vi "LINC Parse Text Command.vi"(8 "error in (no error)":errorcluster, 9 "string command":string, 10 "target name":string) -> (0 "error out":errorcluster, 1 "member data":string[](array[string]), 2 "member names":string[](array[string]), 3 "packet name":string, 5 "member types":string[](array[string]))   [LabVIEW 2018, in "STEPkgDriver_LINC.lvlib"]
uses:
  STEPkgDriver_LINC.lvlib
  LINC Global Mode.ctl
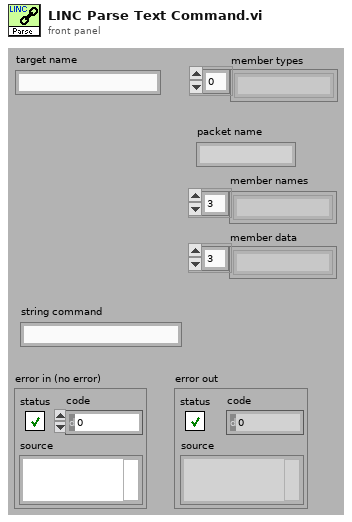
[diagram p1: front panel]
types:
  T1 = typedef "STEPkgDriver_LINC.lvlib/LINC Global Mode.ctl" = enum16{"INIT", "CLEAR", "ADD_PKT_HDR", "ADD_PKT", "GET_PKT_NAMES", "GET_PKT_DESC", "GET_PKT_HDR", "GET_PKT", "SET_PKT", "SET_DATA", "SIM_EN", "SIM_DS"}
  T2 = typedef "STEPkgDriver_LINC.lvlib/LINC Format Prototype.ctl" = cluster{"type":string, "bit offset":i32, "bit size":i32, "format":string, "unit":string, "description":string, "state values":i64[], "states":string[], "max":string, "min":string, "default":string, "array":bool, "bit element size":i32, "poly bound":dbl[], "poly scale":cluster{"coefficients":dbl[]}[], "labview size":i32, "simulate":bool, "ID":bool, "required":bool}
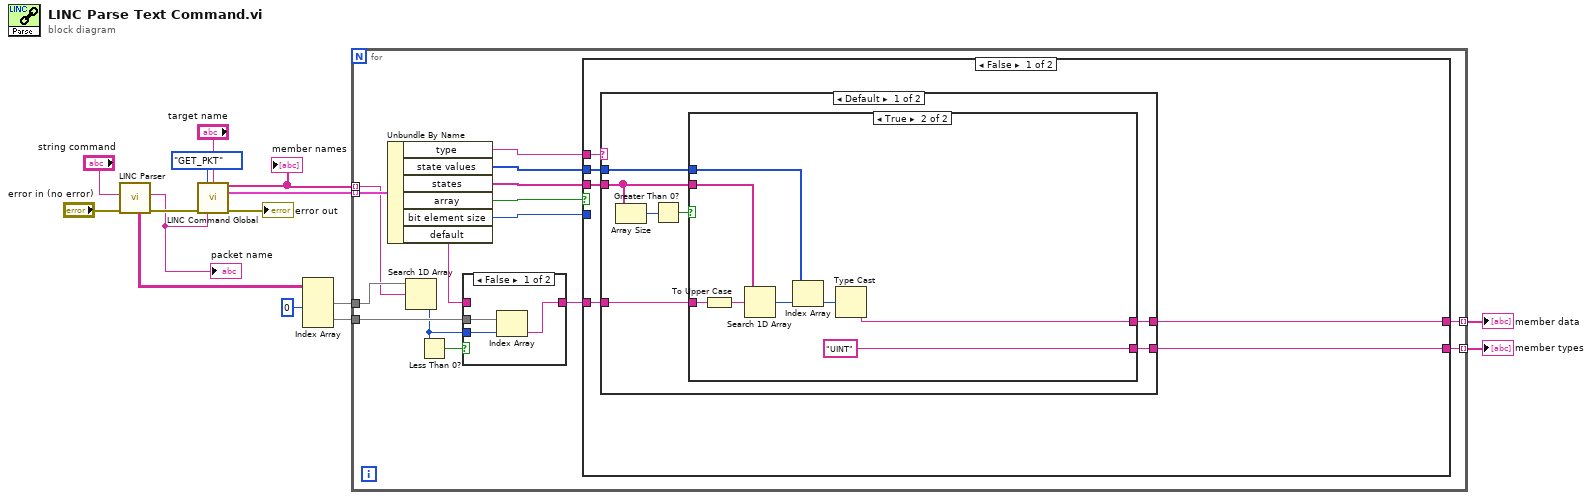
[diagram p0: block diagram]
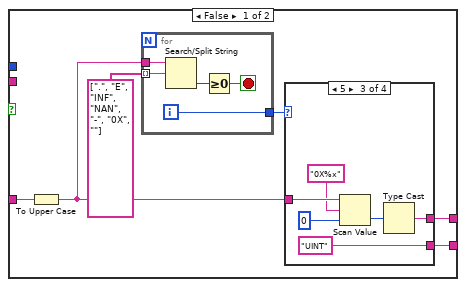
[diagram p3: hidden frame]
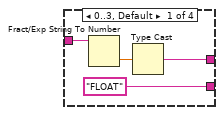
[diagram p4: hidden frame]
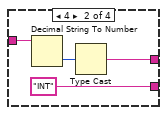
[diagram p5: hidden frame]
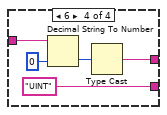
[diagram p6: hidden frame]
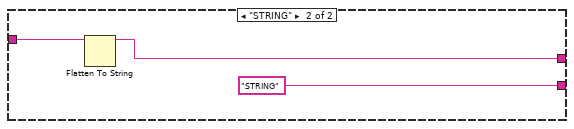
[diagram p7: hidden frame]
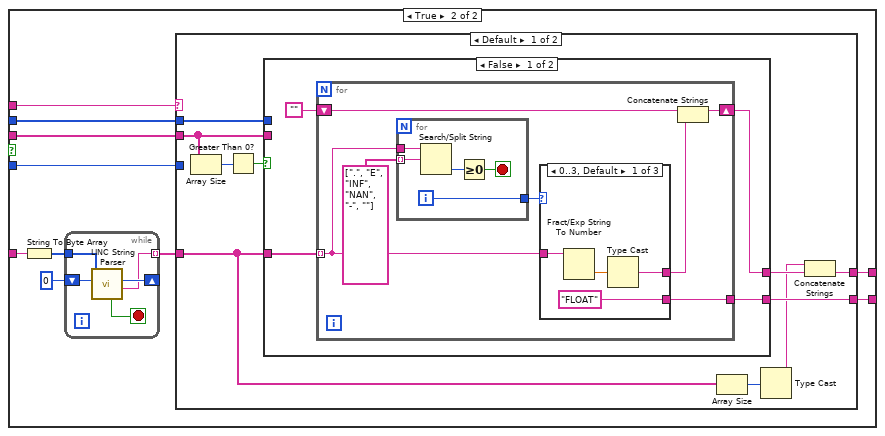
[diagram p8: hidden frame]
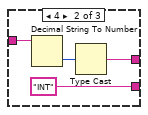
[diagram p9: hidden frame]
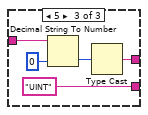
[diagram p10: hidden frame]
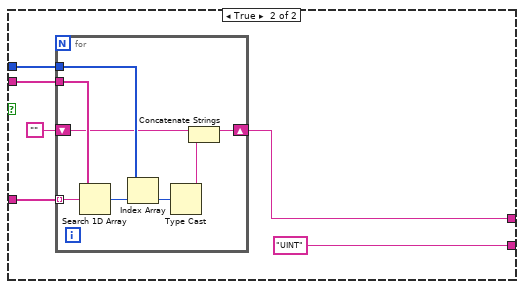
[diagram p11: hidden frame]
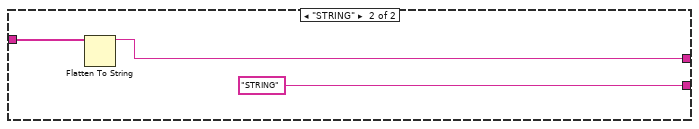
[diagram p12: hidden frame]
diagram:
  n1 = call "LINC Parser.vi"("error in (no error)"="error in (no error)", "command in"="string command") -> ("error out"=w4:errorcluster, "command"=w1:string, "command arguments"=w9:string[][])  [unwired: 7 in]
  "packet name" <- w1
  n2 = call "LINC Command Global.vi"("mode"=LINC_Global_Mode."GET_PKT", "target name"="target name", "error in (no error)"=w4, "packet name"=w1) -> ("values out"=w12:string[], "item formats out"=w11:T2[], "error out"=→"error out":errorcluster)  [unwired: 7 in, 2 out]
  "member names" <- w12
  n3 = Index Array(array=w9, index (col) #1=0 ("index")) -> (element #1=w8:string[], element #2=w7:string[])  [unwired: 3 in]
  n4 = for {
    tunnel: w11 -> [w26] mode=indexing
    tunnel: w12 -> [w24] mode=indexing
    tunnel: w8 -> [w25]
    tunnel: w7 -> [w23]
    tunnel: [w21] -> w6 mode=indexing
    tunnel: [w20] -> w5 mode=indexing
    n5 = Unbundle By Name(w26) -> ("type"=w29:string, "state values"=w28:i64[], "states"=w27:string[], "array"=w30:bool, "bit element size"=w16:i32, "default"=w17:string)
    n6 = Search 1D Array(1D array=w25, element=w24) -> (index of element=w19:i32)  [unwired: 1 in]
    n7 = Less Than 0?(x=w19) -> (x < 0?=w18:bool)
    n8 = case shown="False" w18 {
      tunnel: w23 -> [w33 _]
      tunnel: [w32 w34] -> w22
      tunnel: w19 -> [w31 _]
      tunnel: w17 -> [_ w34]
      frame False {
        n9 = Index Array(array=w33, index=w31) -> (element=w32:string)
      }
      frame True {
      }
    }
    n10 = case shown="False" w30 {
      tunnel: w29 -> [w40 w98]
      tunnel: w22 -> [w39 w93]
      tunnel: w28 -> [w38 w97]
      tunnel: w27 -> [w37 w96]
      tunnel: [w36 w90] -> w20
      tunnel: [w35 w89] -> w21
      tunnel: w16 -> [_ w92]
      frame False {
        n11 = case shown="Default" w40 {
          tunnel: w39 -> [w46 w87]
          tunnel: w38 -> [w43 _]
          tunnel: w37 -> [w44 _]
          tunnel: [w41 w86] -> w36
          tunnel: [w42 "STRING" ("new element/subarray")] -> w35
          frame Default {
            n12 = Array Size(array=w44) -> (size(s)=w47:i32)
            n13 = Greater Than 0?(x=w47) -> (x > 0?=w45:bool)
            n14 = case shown="True" w45 {
              tunnel: w46 -> [w50 w84]
              tunnel: w44 -> [_ w85]
              tunnel: w43 -> [_ w83]
              tunnel: [w49 w80] -> w41
              tunnel: [w51 "UINT" ("new element/subarray")] -> w42
              frame False {
                n15 = To Upper Case(1:w50) -> (0:w48:string)
                n16 = for {
                  tunnel: w48 -> [w77]
                  tunnel: string[] [".", "E", "INF", "NAN", "-", "0X", ""] ("operators (none)") -> [w76] mode=indexing
                  tunnel: [w73] -> w52
                  i -> [w73]
                  stop <- w75 stop-if-true
                  n17 = Search/Split String(string=w77, search string/char (-)=w76) -> (offset of match=w74:i32)  [unwired: 1 in, 2 out]
                  n18 = Greater Or Equal To 0?(x=w74) -> (x >= 0?=w75:bool)
                }
                n19 = case shown="5" w52 {
                  tunnel: ["FLOAT" "INT" "UINT" "UINT"] -> w51
                  tunnel: w48 -> [w56 w59 w65 w70]
                  tunnel: [w54 w58 w64 w69] -> w49
                  frame 0..3, Default {
                    n20 = Fract/Exp String To Number(string=w56) -> (number=w55:dbl)  [unwired: 3 in, 1 out]
                    n21 = Type Cast(x=w55) -> (*(type *) &x=w54:string)  [unwired: 1 in]
                  }
                  frame 4 {
                    n22 = Decimal String To Number(string=w59) -> (number=w60:i32)  [unwired: 2 in, 1 out]
                    n23 = Type Cast(x=w60) -> (*(type *) &x=w58:string)  [unwired: 1 in]
                  }
                  frame 5 {
                    n24 = Scan Value(string=w65, format string="0X%x", default (0 dbl)=u32 0 ("default (0 I32)")) -> (value=w66:u32)  [unwired: 1 out]
                    n25 = Type Cast(x=w66) -> (*(type *) &x=w64:string)  [unwired: 1 in]
                  }
                  frame 6 {
                    n26 = Decimal String To Number(string=w70, default (0L)=u32 0 ("default (0 I32)")) -> (number=w71:u32)  [unwired: 1 in, 1 out]
                    n27 = Type Cast(x=w71) -> (*(type *) &x=w69:string)  [unwired: 1 in]
                  }
                }
              }
              frame True {
                n28 = To Upper Case(1:w84) -> (0:w78:string)
                n29 = Search 1D Array(1D array=w85, element=w78) -> (index of element=w82:i32)  [unwired: 1 in]
                n30 = Index Array(array=w83, index=w82) -> (element=w81:i64)
                n31 = Type Cast(x=w81) -> (*(type *) &x=w80:string)  [unwired: 1 in]
              }
            }
          }
          frame "STRING" {
            n32 = Flatten To String(anything=w87) -> (data string=w86:string)  [unwired: 3 in, 2 out]
          }
        }
      }
      frame True {
        n33 = String To Byte Array(string=w93) -> (unsigned byte array=w95:u8[])
        n34 = while {
          shift-right: [w101] -> _
          shift-left: 0 ("index out") -> [w102]
          tunnel: w95 -> [w103]
          tunnel: [w99] -> w91 mode=indexing
          stop <- w100 stop-if-true
          n35 = call "LINC String Parser.vi"("index in"=w102, "string in"=w103) -> ("string found"=w99:string, "index out"=w101:i32, "end"=w100:bool)  [unwired: 5 in, 2 out]
        }
        n36 = case shown="Default" w98 {
          tunnel: w91 -> [w108 w158]
          tunnel: w97 -> [w110 _]
          tunnel: w96 -> [w111 _]
          tunnel: [w104 w157] -> w90
          tunnel: [w109 "STRING" ("new element/subarray")] -> w89
          tunnel: w92 -> [_ _]
          frame Default {
            n37 = Array Size(array=w111) -> (size(s)=w113:i32)
            n38 = Greater Than 0?(x=w113) -> (x > 0?=w112:bool)
            n39 = case shown="False" w112 {
              tunnel: w108 -> [w116 w147]
              tunnel: w111 -> [_ w148]
              tunnel: w110 -> [_ w146]
              tunnel: [w114 w143] -> w106
              tunnel: [w117 "UINT" ("new element/subarray")] -> w109
              frame False {
                n40 = for {
                  tunnel: [w122] -> w117
                  tunnel: w116 -> [w121] mode=indexing
                  shift-right: [w119] -> w114
                  shift-left: "" -> [w120]
                  n41 = for {
                    tunnel: w121 -> [w142]
                    tunnel: string[] [".", "E", "INF", "NAN", "-", ""] ("operators (none)") -> [w141] mode=indexing
                    tunnel: [w138] -> w123
                    i -> [w138]
                    stop <- w140 stop-if-true
                    n42 = Search/Split String(string=w142, search string/char (-)=w141) -> (offset of match=w139:i32)  [unwired: 1 in, 2 out]
                    n43 = Greater Or Equal To 0?(x=w139) -> (x >= 0?=w140:bool)
                  }
                  n44 = case shown="0..3, Default" w123 {
                    tunnel: ["FLOAT" "INT" "UINT"] -> w122
                    tunnel: w121 -> [w127 w130 w135]
                    tunnel: [w125 w129 w134] -> w118
                    frame 0..3, Default {
                      n45 = Fract/Exp String To Number(string=w127) -> (number=w126:dbl)  [unwired: 3 in, 1 out]
                      n46 = Type Cast(x=w126) -> (*(type *) &x=w125:string)  [unwired: 1 in]
                    }
                    frame 4 {
                      n47 = Decimal String To Number(string=w130) -> (number=w131:i32)  [unwired: 2 in, 1 out]
                      n48 = Type Cast(x=w131) -> (*(type *) &x=w129:string)  [unwired: 1 in]
                    }
                    frame 5 {
                      n49 = Decimal String To Number(string=w135, default (0L)=u32 0 ("default (0 I32)")) -> (number=w136:u32)  [unwired: 1 in, 1 out]
                      n50 = Type Cast(x=w136) -> (*(type *) &x=w134:string)  [unwired: 1 in]
                    }
                  }
                  n51 = Concatenate Strings(w120, w118) -> (w119:string)
                }
              }
              frame True {
                n52 = for {
                  tunnel: w148 -> [w156]
                  tunnel: w147 -> [w155] mode=indexing
                  tunnel: w146 -> [w154]
                  shift-right: [w150] -> w143
                  shift-left: "" -> [w151]
                  n53 = Search 1D Array(1D array=w156, element=w155) -> (index of element=w153:i32)  [unwired: 1 in]
                  n54 = Index Array(array=w154, index=w153) -> (element=w152:i64)
                  n55 = Type Cast(x=w152) -> (*(type *) &x=w149:string)  [unwired: 1 in]
                  n56 = Concatenate Strings(w151, w149) -> (w150:string)
                }
              }
            }
            n57 = Array Size(array=w108) -> (size(s)=w107:i32)
            n58 = Type Cast(x=w107) -> (*(type *) &x=w105:string)  [unwired: 1 in]
            n59 = Concatenate Strings(w105, w106) -> (w104:string)
          }
          frame "STRING" {
            n60 = Flatten To String(anything=w158) -> (data string=w157:string)  [unwired: 3 in, 2 out]
          }
        }
      }
    }
  }
  "member data" <- w5
  "member types" <- w6
